vi "DCPower_Reconfig_byChannel.vi"(2 "error in (no error)":errorcluster, 3 "DCPower_ToggleIndex":i32[](array[numeric]), 4 "DCPower_byChannel in 2":T1(array[cluster])) -> (0 "error out":errorcluster, 1 "DCPower_byChannel out":T1(array[cluster]))   [LabVIEW 2019]
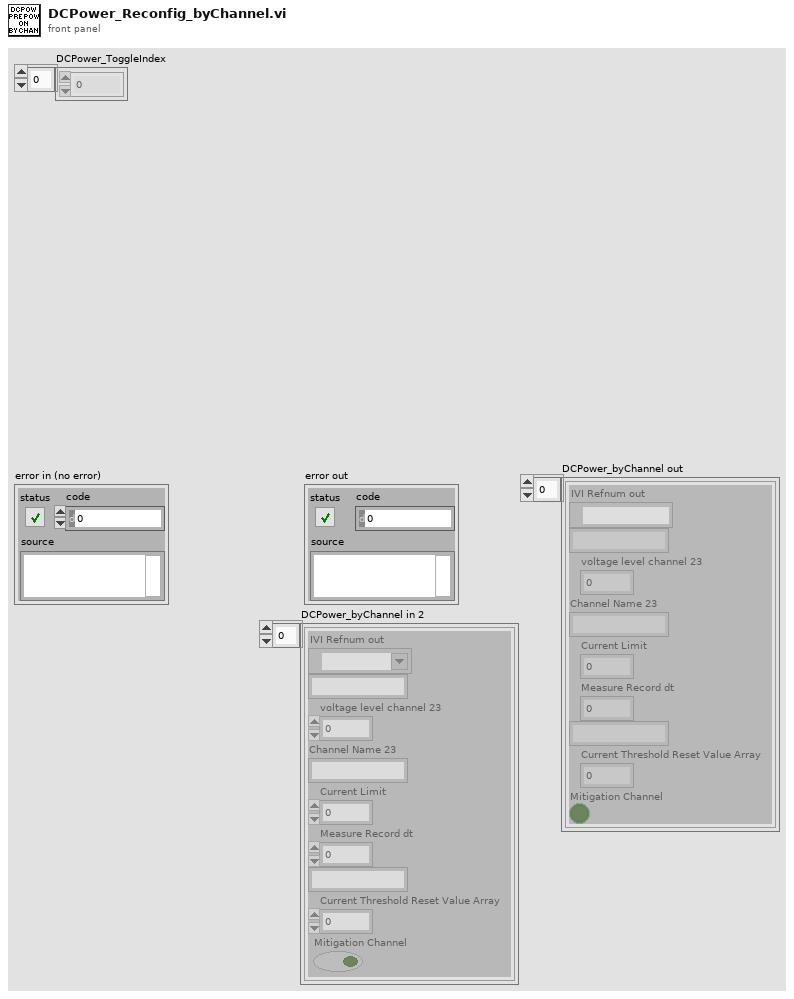
[diagram p1: front panel]
types:
  T1 = cluster{"IVI Refnum out":refnum<k15>, string, "voltage level channel 23":dbl, "Channel Name 23":string, "Current Limit":dbl, "Measure Record dt":dbl, string, "Current Threshold Reset Value Array":dbl, "Mitigation Channel":bool}[]
  T2 = cluster{"IVI Refnum out":refnum<k15>, string, "voltage level channel 23":dbl, "Channel Name 23":string, "Current Limit":dbl, "Measure Record dt":dbl, string, "Current Threshold Reset Value Array":dbl, "Mitigation Channel":bool}
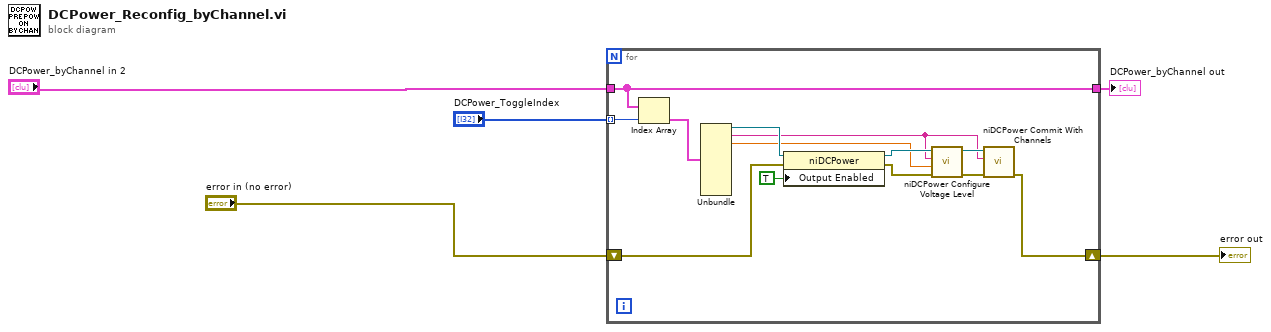
[diagram p0: block diagram]
diagram:
  n1 = for {
    shift-right: [w7] -> w5
    shift-left: "error in (no error)" -> [w17]
    tunnel: "DCPower_byChannel in 2" -> [w6]
    tunnel: "DCPower_ToggleIndex" -> [w15] mode=indexing
    tunnel: [w6] -> w1
    n2 = Index Array(array=w6, index=w15) -> (element=w14:T2)
    n3 = Unbundle(w14) -> ("IVI Refnum out"=w18:refnum<k15>, w8:string, "voltage level channel 23"=w9:dbl)  [unwired: 6 out]
    n4 = property class="niDCPower"(reference=w18, error in=w17, "Output Enabled"=TRUE ("Source:Output Enabled")) -> (reference out=w10:refnum<k15>, error out=w11:errorcluster)
    n5 = call <instrlib>:"niDCPower Configure Voltage Level.vi"("error in (no error)"=w11, "voltage level"=w9, "channel name"=w8, "instrument handle"=w10) -> ("error out"=w13:errorcluster, "instrument handle out"=w12:refnum<k15>)  [unwired: 6 in]
    n6 = call <instrlib>:"niDCPower Commit With Channels.vi"("error in (no error)"=w13, "channel name"=w8, "instrument handle"=w12) -> ("error out"=w7:errorcluster)  [unwired: 7 in, 1 out]
  }
  "error out" <- w5
  "DCPower_byChannel out" <- w1
